vi "Get Next UUT.vi"(11 "Number of UUTs":u32) -> (2 "End of List":bool, 3 "next UUT":u16)   [LabVIEW 2013]
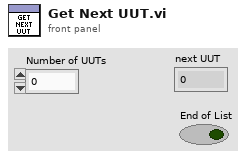
[diagram p1: front panel]
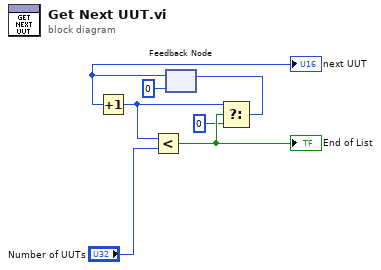
[diagram p0: block diagram]
diagram:
  n1 = feedback #1(u16 0 ("f")) -> (w7:u16)
  "next UUT" <- w7
  n2 = Increment(x=w7) -> (x+1=w3:u16)
  n3 = Less?(x=w3, y="Number of UUTs") -> (x < y?=w6:bool)
  "End of List" <- w6
  n4 = Select(t=w3, s=w6, f=u16 0) -> (s? t:f=w5:u16)
  n5 = feedback-in #1(w5) -> ()
